vi "Reef Align Command_wrapper.vi"() -> ()   [LabVIEW 2023]
uses:
  <vilib>/Rock Robotics/WPI/Framework/Command Status Info.ctl
  <vilib>/Rock Robotics/WPI/Framework/Completion Status.ctl
  <vilib>/Rock Robotics/WPI/Framework/Completion Notifier.ctl
  Implementation/Drive Setpoints.ctl
  Implementation/Drive Operations.ctl
  swerve/Type Definitions/Data/Robot Velocities.ctl
panel:
  out "Command Timing":cluster{"Start Time (ms)":u32, "Iterations":i32}
  out "SubSystem Data 2":T1
  out "Command Info Out":T4
  in  "Aligning?":bool
  in  "SubSystem Data":T1={"Operation"=enum."Reef Align", "Robot Velocities"={"X Velocity"=0.0, "Y Velocity"=0.0, "Rotational \nVelocity"=0.0}, "Auto Data"={"Auto Velocities"=[], "Auto Positions"=[], "Auto Commands"=[], "Zero Velocity?"=[]}, "Left side"=FALSE, "Angle Align"=FALSE, "Tag ID"=0}
  in  "Description":string
  in  "Command Info In":T4
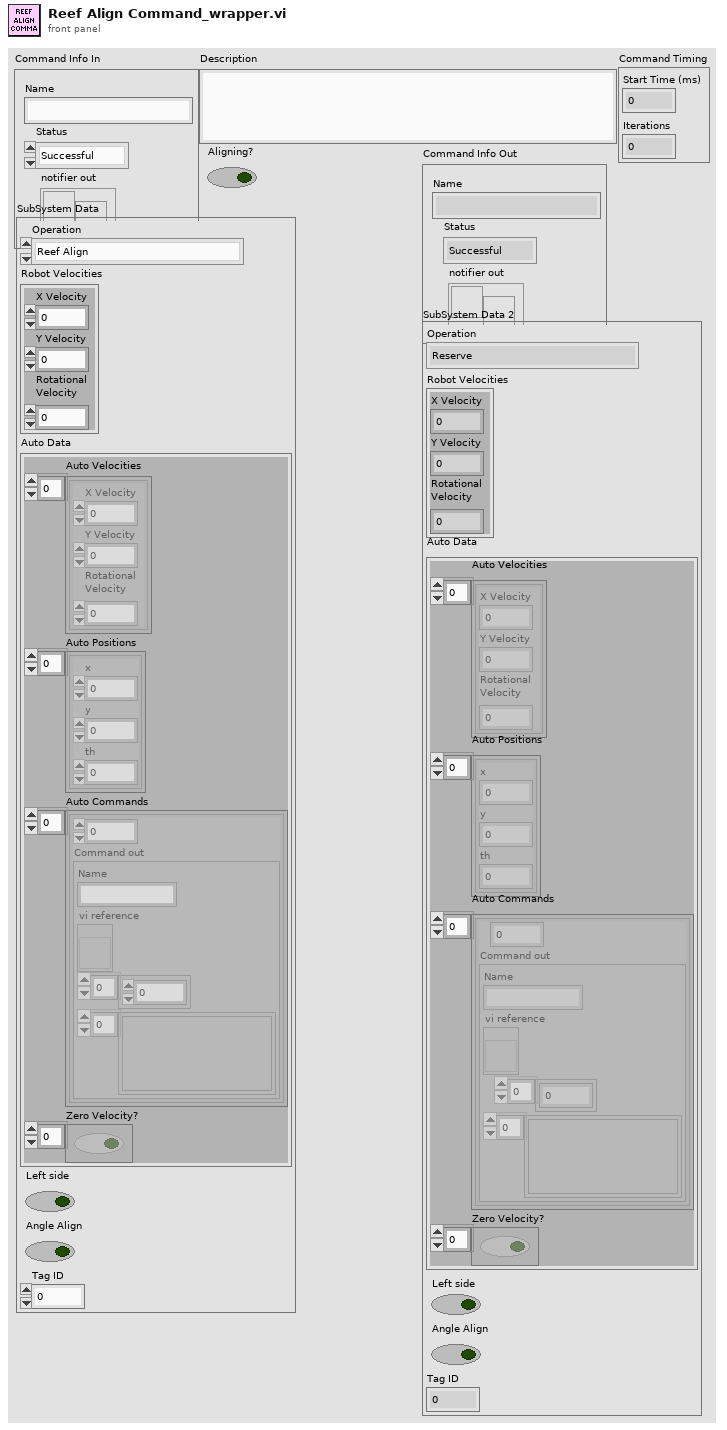
[diagram p1: front panel]
types:
  T1 = typedef "Drive Setpoints.ctl" = cluster{"Operation":T2, "Robot Velocities":T3, "Auto Data":cluster{"Auto Velocities":T3[], "Auto Positions":cluster{"x":dbl, "y":dbl, "th":dbl}[], "Auto Commands":cluster{dbl, "Command out":cluster{"Name":string, "vi reference":refnum<vi>, i32[], variant[]}}[], "Zero Velocity?":bool[]}, "Left side":bool, "Angle Align":bool, "Tag ID":i32}
  T2 = typedef "Drive Operations.ctl" = enum16{"Reserve", "Read Current", "Immediate", "Calibrate", "Reef Align", "Auto"}
  T3 = typedef "Robot Velocities.ctl" = cluster{"X Velocity":dbl, "Y Velocity":dbl, "Rotational \nVelocity":dbl}
  T4 = typedef "Command Status Info.ctl" = cluster{"Name":string, "Status":T5, "notifier out":T6}
  T5 = typedef "Completion Status.ctl" = enum16{"Successful", "Aborted", "Incomplete"}
  T6 = typedef "Completion Notifier.ctl" = refnum<notifier>
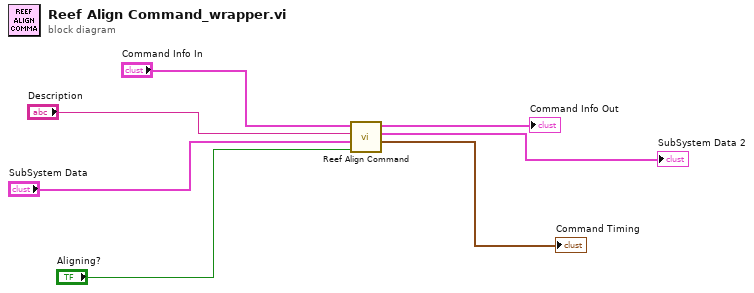
[diagram p0: block diagram]
diagram:
  n1 = call "Reef Align Command.vi"("Aligning?"="Aligning?", "SubSystem Data"="SubSystem Data", "Description"="Description", "Command Info In"="Command Info In") -> ("Command Timing"=→"Command Timing":cluster{"Start Time (ms)":u32, "Iterations":i32}, "SubSystem Data 2"=→"SubSystem Data 2":T1, "Command Info Out"=→"Command Info Out":T4)  [unwired: 5 in]
